vi "Initialize.vi"(7 "Channel Name":string="Setpoint.ch%d.SP", 8 "error in":errorcluster, 9 "Number of Channels":u32=1, 10 "Instance Name":string="PluginName", 11 "Voltage Gradient in":refnum<class "Voltage Gradient.lvclass">) -> (0 "error out":errorcluster, 3 "Voltage Gradient out":refnum<class "Voltage Gradient.lvclass">)   [LabVIEW 2023, in "Voltage Gradient.lvclass"]
uses:
  Voltage Gradient.lvclass
  Voltage Gradient.lvclass/Voltage Gradient.ctl
  Parents/Gradient/Gradient.lvclass
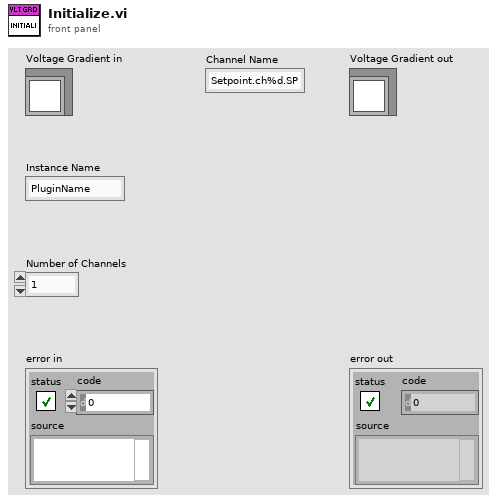
[diagram p1: front panel]
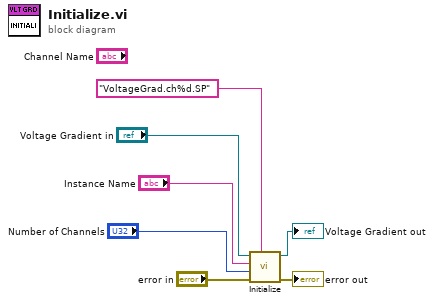
[diagram p0: block diagram]
diagram:
  n1 = call-parent "Initialize.vi"("Channel Name"="VoltageGrad.ch%d.SP" ("ChannelName"), "error in"="error in", "Number of Channels"="Number of Channels", "Instance Name"="Instance Name", "Gradient in"="Voltage Gradient in") -> ("error out"=→"error out":errorcluster, "Gradient out"=→"Voltage Gradient out":refnum<class "Voltage Gradient.lvclass">)  [unwired: 5 in]
